vi "Update test_serialize_deserialize.vi"(8 "error in (no error)":errorcluster, 11 "Path to Library":path) -> (0 "error out":errorcluster)   [LabVIEW 2020]
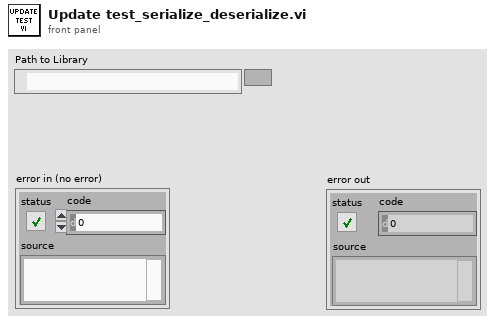
[diagram p1: front panel]
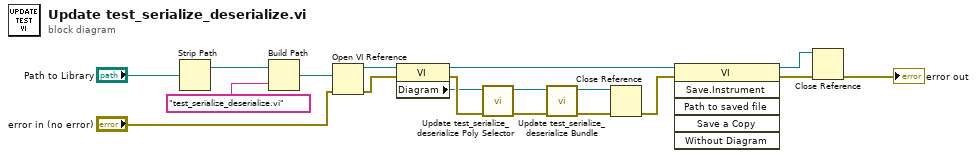
[diagram p0: block diagram]
diagram:
  n1 = Strip Path(path="Path to Library") -> (stripped path=w1:path)  [unwired: 1 out]
  n2 = Build Path(base path=w1, name or relative path="test_serialize_deserialize.vi" ("pattern")) -> (appended path=w16:path)
  n3 = Open VI Reference(vi path=w16, error in (no error)="error in (no error)") -> (vi reference=w5:refnum<vi>, error out=w6:errorcluster)  [unwired: 4 in]
  n4 = property class="VI"(reference=w5, error in=w6) -> (reference out=w9:refnum<vi>, error out=w18:errorcluster, "Diagram"=w15:refnum<vi>)
  n5 = call "Update test_serialize_deserialize Poly Selector.vi"("error in (no error)"=w18, "Diagram in"=w15) -> ("error out"=w13:errorcluster, "Diagram out"=w14:refnum<vi>)  [unwired: 8 in]
  n6 = call "Update test_serialize_deserialize Bundle.vi"("error in (no error)"=w13, "Diagram in"=w14) -> ("error out"=w11:errorcluster, "Diagram out"=w12:refnum<vi>)  [unwired: 8 in]
  n7 = Close Reference(reference=w12, error in (no error)=w11) -> (error out=w10:errorcluster)
  n8 = invoke class="VI" method="Save.Instrument"(reference=w9, error in=w10) -> (reference out=w7:refnum<vi>, error out=w8:errorcluster)  [unwired: 4 in, 4 out]
  n9 = Close Reference(reference=w7, error in (no error)=w8) -> (error out=→"error out":errorcluster)
